vi "Read SM1000.vi"(8 "error in (no error)":errorcluster, 11 "HC-Main in":refnum<class "MC-Main.lvclass">) -> (0 "error out":errorcluster, 2 "Object reference":T1, 3 "HC-Main out":refnum<class "MC-Main.lvclass">)   [LabVIEW 2013, in "MaterialCharacterization.lvlib" / "MC-Main.lvclass"]
uses:
  MC-Main.lvclass
  SM1000/Object-reference.ctl
  SM1000/MC-SM1000.lvclass
  MC-Main.lvclass/MC-Main.ctl
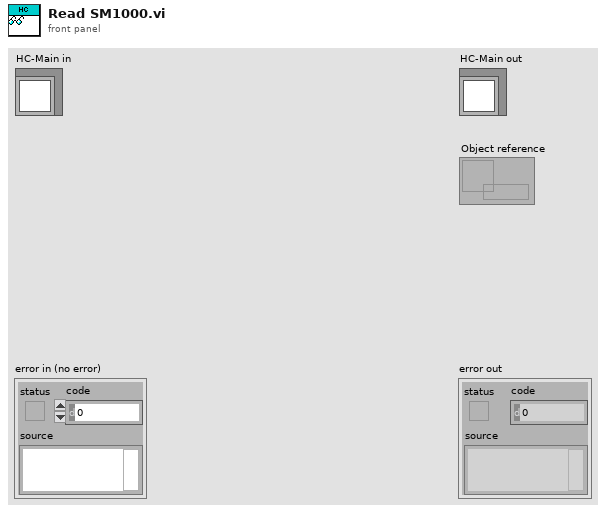
[diagram p1: front panel]
types:
  T1 = typedef "MaterialCharacterization.lvlib/MC-SM1000.lvclass/Object-reference.ctl" = refnum<data-value>
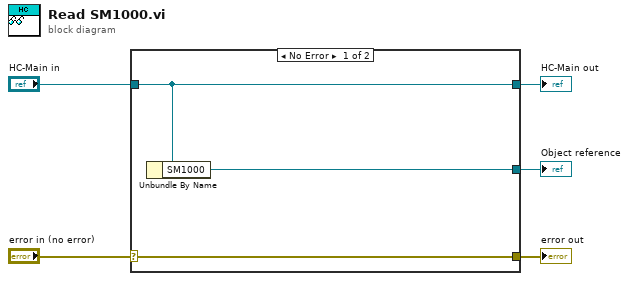
[diagram p0: block diagram]
diagram:
  n1 = case shown="No Error" "error in (no error)" {
    selector: "error in (no error)" -> [w8 w9]
    tunnel: [w8 w9] -> w4
    tunnel: [w7 w10] -> w2
    tunnel: "HC-Main in" -> [w7 w10]
    tunnel: [w6 _] -> w1
    frame No Error {
      n2 = Unbundle By Name(w7) -> ("SM1000"=w6:T1)
    }
    frame Error {
    }
  }
  "error out" <- w4
  "HC-Main out" <- w2
  "Object reference" <- w1
